vi "Do.vi"(7 "Mediated Asynchronous Actor":refnum<class "Mediated Asynchronous Actor.lvclass">, 8 "error in (no error)":errorcluster, 11 "Add Connected Client to WSserver Msg in":refnum<class "Add Connected Client to WSserver Msg.lvclass">) -> (0 "error out":errorcluster, 3 "Add Connected Client to WSserver Msg out":refnum<class "Add Connected Client to WSserver Msg.lvclass">, 5 "Mediated Asynchronous Actor out":refnum<class "Mediated Asynchronous Actor.lvclass">)   [LabVIEW 2016, in "WebSocket Networking.lvlib" / "Add Connected Client to WSserver Msg.lvclass"]
doc: "--\nCopyright © 2017 Composed SystemsI All rights reserved.\n\nAuthor: Jon McBee <jon.mcbee@composed.io>\n\nThis library is provided \"AS IS\" ,WITHOUT WARRANTIES OR\nCONDITIONS OF ANY KIND, either express or implied.\n\nComposed Systems -- composed.io\n\nStream 0.0.1.1\nJon McBee - Composed Systems\nCopyright (c) 2017, Composed Systems"
uses:
  <userlib>/Common Components/WebSocket Networking/WS Server Msgs/Add Connected Client to WSserver Msg/Add Connected Client to WSserver Msg.lvclass
  <userlib>/Composed Systems/Stream/Mediator/Classes/Mediated Asynchronous Actor/Mediated Asynchronous Actor.lvclass
  <userlib>/Common Components/WebSocket Networking/WS Server/WS Server.lvclass
  C:/Program Files (x86)/National Instruments/LabVIEW 2016/user.lib/Composed Systems/Stream/Mediator/Classes/Mediated Asynchronous Actor/Mediated Asynchronous Actor.lvclass
  <userlib>/Common Components/WebSocket Networking/WS Server Msgs/Add Connected Client to WSserver Msg/Add Connected Client to WSserver Msg.lvclass/Add Connected Client to WSserver Msg.ctl
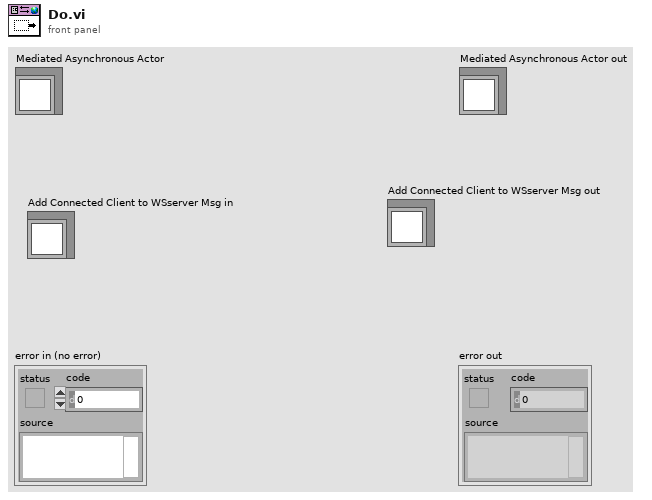
[diagram p1: front panel]
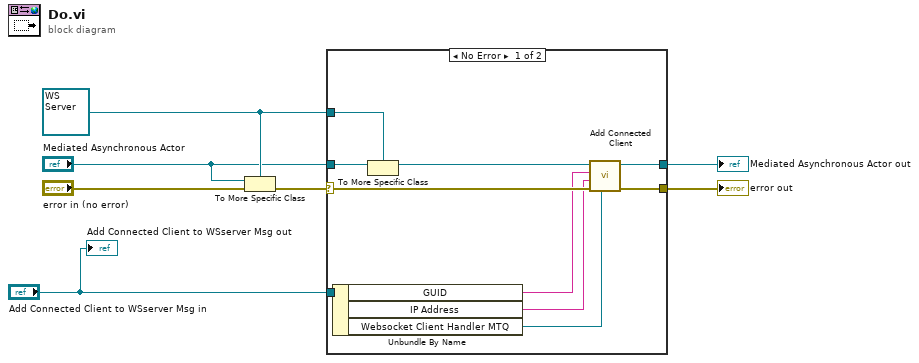
[diagram p0: block diagram]
diagram:
  w5 = refnum<class "WS Server.lvclass"> refnum ("Websocket Server.lvclass")
  n1 = To More Specific Class(target class=w5, reference="Mediated Asynchronous Actor", error in="error in (no error)") -> (error out=w7:errorcluster)  [unwired: 1 out]
  n2 = case shown="No Error" w7 {
    selector: w7 -> [w12 w18]
    tunnel: w5 -> [w17 _]
    tunnel: "Mediated Asynchronous Actor" -> [w16 w19]
    tunnel: "Add Connected Client to WSserver Msg in" -> [w15 _]
    tunnel: [w13 w19] -> w3
    tunnel: [w11 w18] -> w2
    frame No Error {
      n3 = Unbundle By Name(w15) -> ("GUID"=w10:string, "IP Address"=w9:string, "Websocket Client Handler MTQ"=w8:refnum<class "Message Transport Queue.lvclass">)
      n4 = To More Specific Class(target class=w17, reference=w16) -> (specific class reference=w14:refnum<class "WS Server.lvclass">)  [unwired: 1 in, 1 out]
      n5 = call <userlib>:"Add Connected Client.vi"("Websocket Client Handler MTQ"=w8, "error in (no error)"=w12, "IP"=w9, "GUID"=w10, "Websocket Server in"=w14) -> ("error out"=w11:errorcluster, "Websocket Server out"=w13:refnum<class "WS Server.lvclass">)  [unwired: 5 in]
    }
    frame Error {
    }
  }
  "error out" <- w2
  "Mediated Asynchronous Actor out" <- w3
  "Add Connected Client to WSserver Msg out" <- "Add Connected Client to WSserver Msg in"
